vi "AB_850_860_Project_SourceItems.vi"(5 "Provider Item":T1, 7 "action":T2, 8 "error in (no error)":errorcluster, 10 "oldBuildObject":T1, 11 "buildObject":T1) -> (0 "error out":errorcluster, 3 "buildObject out":T1)   [LabVIEW 2020]
doc: "Reads and writes the data to the object property bag."
uses:
  <resource>/Framework/Providers/API/ItemRef.ctl
  <vilib>/AppBuilder/RW_Project/AB_RW_Project_PropBag_ArrayAction.ctl
  <vilib>/AppBuilder/AB_Source_Inclusion.ctl
  <vilib>/AppBuilder/RW_Project/AB_RW_Project_PropBag_Action.ctl
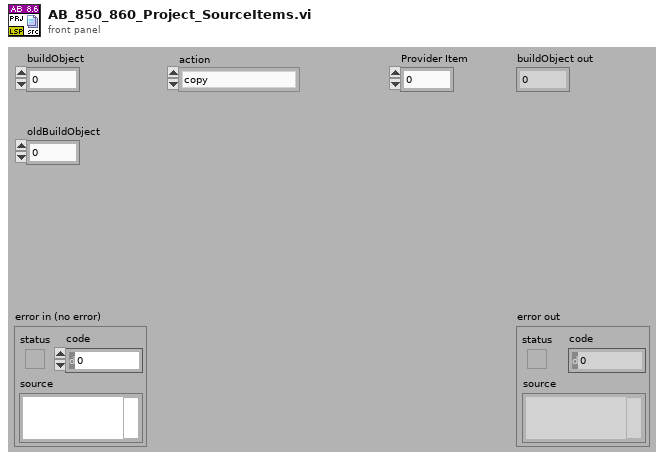
[diagram p1: front panel]
types:
  T1 = typedef "ItemRef.ctl" = u64
  T2 = typedef "AB_RW_Project_PropBag_ArrayAction.ctl" = enum16{"copy", "saveForPrevious", "loadFromPrevious", "clear"}
  T3 = typedef "AB_Source_Inclusion.ctl" = enum16{"IncludeIfReferenced", "Include", "Exclude", "TopLevel"}
  T4 = typedef "AB_RW_Project_PropBag_Action.ctl" = enum16{"read", "write", "clear", "readPrevious", "writePrevious", "clearPrevious"}
  T5 = cluster{"itemID":string, "sourceInclusion":T3, "destinationIndex":i32, "properties":cluster{"sourcePropertyType":enum16{"Remove block diagram", "Remove front panel", "Password", "Window has title bar", "Show menu bar", "Show vertical scroll bar", "Show horizontal scroll bar", "Show toolbar", "Show Abort button", "Show fp when called", "Window behavior", "Allow user to close window", "Window run-time position", "Run when opened", "Allow debugging", "Auto error handling", "Generate guard code", "Use stack variables", "Expression folding", "Integer only", "Inline subVI"}, "value":variant}[], "newName":string, "lvfile":bool}
  T6 = cluster{"applyInclusion":bool, "applyDestination":bool, "applyProperties":bool, "applyPassword":bool, "applyPrefix":bool, "applySaveSetttings":bool}
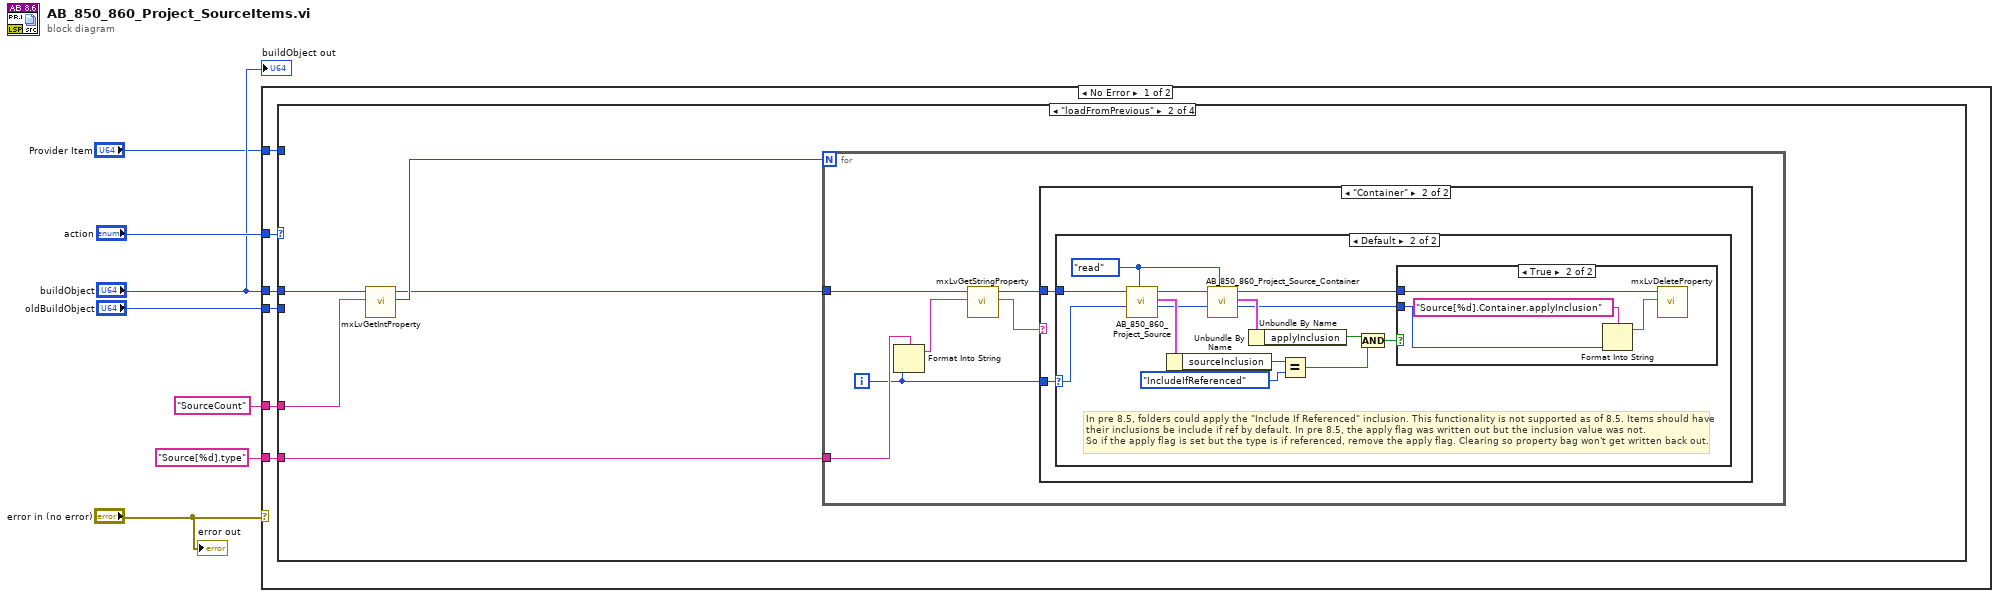
[diagram p0: block diagram]
diagram:
  n1 = case shown="No Error" "error in (no error)" {
    tunnel: "action" -> [w13 _]
    tunnel: "buildObject" -> [w12 _]
    tunnel: "SourceCount" -> [w11 _]
    tunnel: "Source[%d].type" -> [w10 _]
    tunnel: "oldBuildObject" -> [w9 _]
    tunnel: "Provider Item" -> [w8 _]
    frame No Error {
      n2 = case shown="\"loadFromPrevious\"" w13 {
        tunnel: w12 -> [_ w18 _ _]
        tunnel: w11 -> [_ w15 _ _]
        tunnel: w10 -> [_ w17 _ _]
        tunnel: w9 -> [_ _ _ _]
        tunnel: w8 -> [_ _ _ _]
        frame "copy" {
        }
        frame "loadFromPrevious" {
          n3 = call <resource>:"mxLvGetIntProperty.vi"("Tag"=w15, "Item"=w18) -> ("Value"=w16:i32, "Item"=w14:T1)  [unwired: 1 in, 7 out]
          n4 = for {
            N: w16 -> [_]
            tunnel: w17 -> [w24]
            tunnel: w14 -> [w22]
            i -> [w23]
            n5 = Format Into String(format string=w24, w23) -> (resulting string=w21:string)  [unwired: 2 in, 1 out]
            n6 = call <resource>:"mxLvGetStringProperty.vi"("Tag"=w21, "Item"=w22) -> ("Value"=w20:string, "Item"=w19:T1)  [unwired: 1 in, 7 out]
            n7 = case shown="\"Container\"" w20 {
              tunnel: w19 -> [_ w26]
              tunnel: w23 -> [_ w25]
              frame Default {
              }
              frame "Container" {
                n8 = case shown="Default" w25 {
                  selector: w25 -> [_ w29]
                  tunnel: w26 -> [_ w40]
                  frame 0 {
                    # "Zero index is dependency node. Don't make any changes to it even though its type is Container."
                  }
                  frame Default {
                    w38 = AB_RW_Project_PropBag_Action."read" ("action")
                    # "In pre 8.5, folders could apply the \"Include If Referenced\" inclusion. This functionality is not supported as of 8.5. Items should have their inclusions be include if ref by default. In pre 8.5, the apply flag was written out but the inclusion value was not. \nSo if the apply flag is set but the type is if referenced, remove the apply flag. Clearing so property bag won't get written back out."
                    n9 = call <vilib>:"AB_850_860_Project_Source.vi"("action"=w38, "index in"=w29, "buildObject"=w40) -> ("index out"=w28:i32, "dataSource out"=w37:T5, "buildObject out"=w39:T1)  [unwired: 5 in, 1 out]
                    n10 = Unbundle By Name(w37) -> ("sourceInclusion"=w35:T3)
                    n11 = call <vilib>:"AB_850_860_Project_Source_Container.vi"("action"=w38, "index in"=w28, "buildObject"=w39) -> ("index out"=w27:i32, "dataSource out"=w30:T6, "buildObject out"=w36:T1)  [unwired: 5 in, 1 out]
                    n12 = Unbundle By Name(w30) -> ("applyInclusion"=w33:bool)
                    n13 = Equal?(x=w35, y=AB_Source_Inclusion."IncludeIfReferenced") -> (x = y?=w32:bool)
                    n14 = And(x=w33, y=w32) -> (x .and. y?=w31:bool)
                    n15 = case shown="True" w31 {
                      tunnel: w36 -> [_ w42]
                      tunnel: w27 -> [_ w43]
                      frame False {
                      }
                      frame True {
                        n16 = Format Into String(format string="Source[%d].Container.applyInclusion", w43) -> (resulting string=w41:string)  [unwired: 2 in, 1 out]
                        n17 = call <resource>:"mxLvDeleteProperty.vi"("Tag"=w41, "Item"=w42) -> ()  [unwired: 1 in, 9 out]
                      }
                    }
                  }
                }
              }
            }
          }
        }
        frame "saveForPrevious" {
        }
        frame "clear" {
        }
      }
    }
    frame Error {
    }
  }
  "error out" <- "error in (no error)"
  "buildObject out" <- "buildObject"
